vi "GearedSixMotorDriveBegin.vi"(0 "Left Rear Motor":T1=enum."Invalid", 1 "Left Middle Motor":T1=enum."Invalid", 2 "Left Front Motor":T1=enum."Invalid", 3 "Right Rear Motor":T1=enum."Invalid", 4 "Right Middle Motor":T1=enum."Invalid", 5 "Right Front Motor":T1=enum."Invalid", 8 "Left Rear Motor Inverted":bool, 9 "error in (no error)":errorcluster, 10 "Left Middle Motor Inverted":bool, 12 "Left Front Motor Inverted":bool, 14 "Right Rear Motor Inverted":bool, 16 "Right Middle Motor Inverted":bool, 18 "Right Front Motor Inverted":bool) -> (19 "error out":errorcluster, 20 "RobotDriveDevRef":T2={"DevStatus"={"status"=FALSE, "code"=0, "source"=""}, "Motors[]"=[], "Square Inputs"=FALSE, "Max Output"=1.0})   [LabVIEW 2014]
uses:
  <vilib>/Rock Robotics/SystemInterfaces/DIO/FPGA_DIOPWMChannel.ctl
  <vilib>/Rock Robotics/WPI/RobotDrive/WPI_RobotDriveDevRef.ctl
  <vilib>/Rock Robotics/WPI/MotorControl/WPI_MotorControlDeviceRef.ctl
  <vilib>/Rock Robotics/WPI/MotorControl/WPI_MotorControlType.ctl
  <vilib>/Rock Robotics/SystemInterfaces/Typedef/FPGA_TypedefDigitalModule.ctl
  <vilib>/Rock Robotics/WPI/PWM/WPI_PWMDeadband.ctl
  <vilib>/Rock Robotics/WPI/CAN/Jaguar/SubVIs/WPI_CANJaguar_ControlMode.ctl
  <vilib>/Rock Robotics/WPI/CAN/TalonSRX/WPI_CANTalonSRX_APIControlMode.ctl
  <vilib>/Rock Robotics/WPI/PWM/WPI_PWMTransform_ConPane.ctl
  <vilib>/Rock Robotics/WPI/SafetyOutput/WPI_SafetyOutputConfigMenu.ctl
  <vilib>/Rock Robotics/WPI/MotorControl/WPI_MotorControlOpenCANJaguar.vi
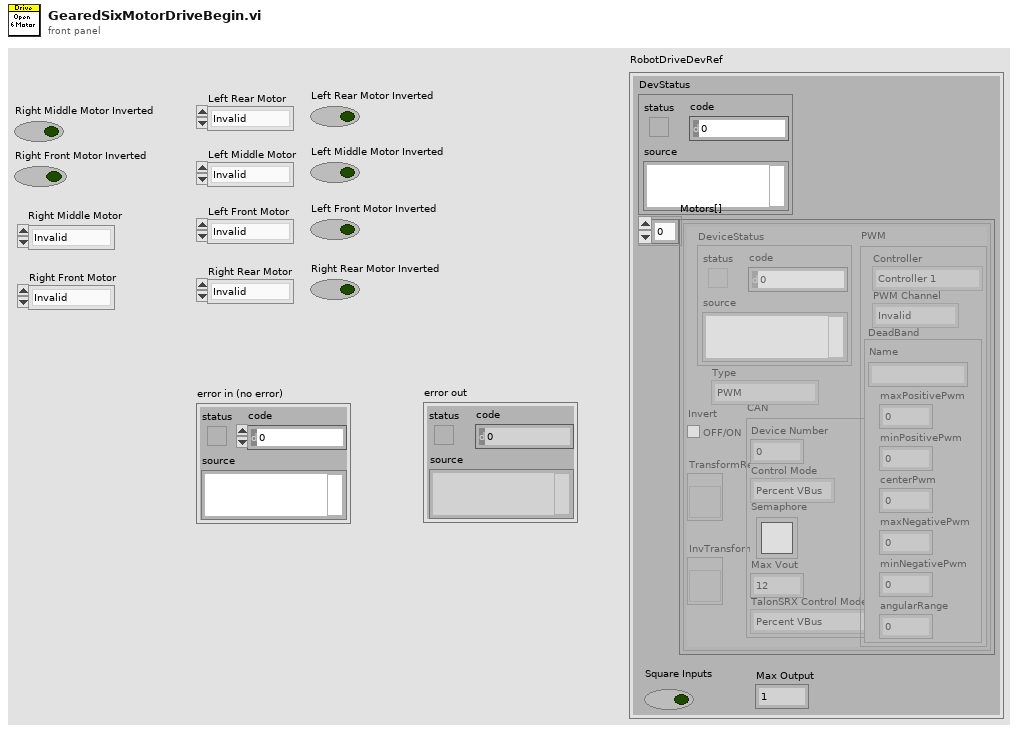
[diagram p1: front panel]
types:
  T1 = typedef "FPGA_DIOPWMChannel.ctl" = enum8{"PWM 0", "PWM 1", "PWM 2", "PWM 3", "PWM 4", "PWM 5", "PWM 6", "PWM 7", "PWM 8", "PWM 9", "PWM MXP 0", "PWM MXP 1", "PWM MXP 2", "PWM MXP 3", "PWM MXP 4", "PWM MXP 5", "PWM MXP 6", "PWM MXP 7", "PWM MXP 8", "PWM MXP 9", "Invalid"}
  T2 = typedef "WPI_RobotDriveDevRef.ctl" = cluster{"DevStatus":errorcluster, "Motors[]":T3[], "Square Inputs":bool, "Max Output":dbl}
  T3 = typedef "WPI_MotorControlDeviceRef.ctl" = cluster{"DeviceStatus":errorcluster, "Type":T4, "PWM":cluster{"Controller":T5, "PWM Channel":T1, "DeadBand":T6}, "CAN":cluster{"Device Number":u8, "Control Mode":T7, "Semaphore":T8, "Max Vout":dbl, "TalonSRX Control Mode":T9}, "Invert":bool, "TransformRef":T10, "InvTransformRef":T10}
  T4 = typedef "WPI_MotorControlType.ctl" = enum16{"PWM", "CAN", "CANTalonSRX"}
  T5 = typedef "FPGA_TypedefDigitalModule.ctl" = enum16{"Controller 1"}
  T6 = typedef "WPI_PWMDeadband.ctl" = cluster{"Name":string, "maxPositivePwm":i32, "minPositivePwm":i32, "centerPwm":i32, "maxNegativePwm":i32, "minNegativePwm":i32, "angularRange":u16}
  T7 = typedef "WPI_CANJaguar_ControlMode.ctl" = enum8{"Percent VBus", "Current", "Speed", "Position", "Voltage"}
  T8 = typedef "Semaphore RefNum" = refnum<k1>
  T9 = typedef "WPI_CANTalonSRX_APIControlMode.ctl" = enum8{"Percent VBus", "Speed", "Position", "Slave", "Unchanged / Invalid"}
  T10 = typedef "WPI_PWMTransform_ConPane.ctl" = refnum<vi>
  T11 = typedef "WPI_SafetyOutputConfigMenu.ctl" = enum16{"Enable", "Disable"}
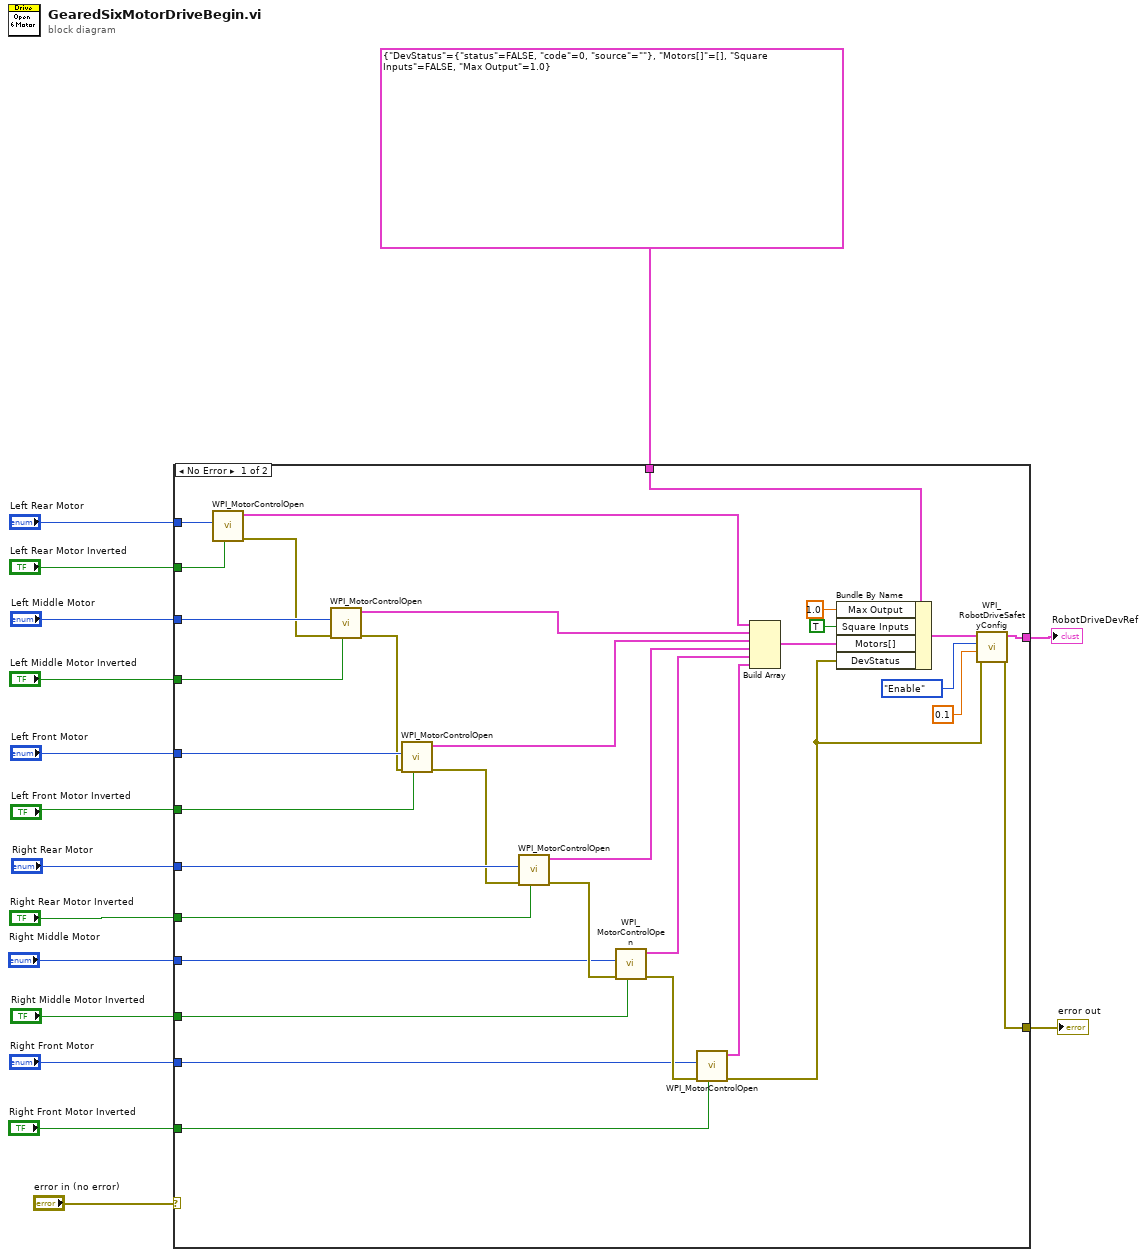
[diagram p0: block diagram]
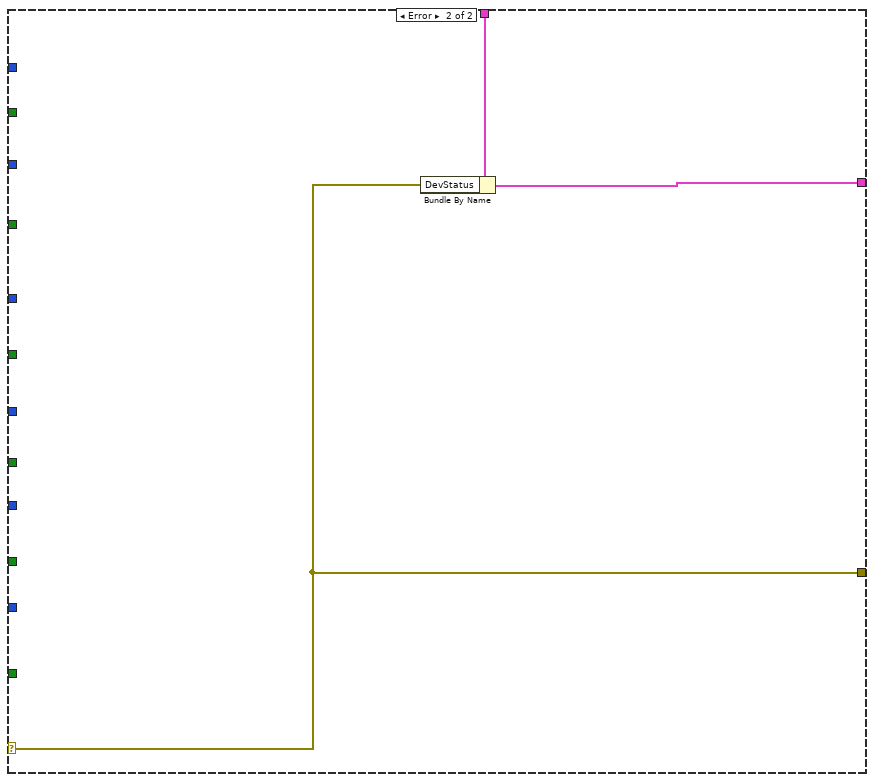
[diagram p2: hidden frame]
diagram:
  n1 = case shown="No Error" "error in (no error)" {
    selector: "error in (no error)" -> [_ w50]
    tunnel: [w30 w51] -> w16
    tunnel: T2 {"DevStatus"={"status"=FALSE, "code"=0, "source"=""}, "Motors[]"=[], "Square Inputs"=FALSE, "Max Output"=1.0} ("RobotDriveDevRef") -> [w49 w52]
    tunnel: "Left Rear Motor" -> [w47 _]
    tunnel: "Right Rear Motor" -> [w44 _]
    tunnel: "Left Front Motor" -> [w45 _]
    tunnel: "Left Middle Motor" -> [w46 _]
    tunnel: "Left Rear Motor Inverted" -> [w36 _]
    tunnel: "Left Middle Motor Inverted" -> [w35 _]
    tunnel: "Right Rear Motor Inverted" -> [w33 _]
    tunnel: "Left Front Motor Inverted" -> [w34 _]
    tunnel: [w31 w50] -> w5
    tunnel: "Right Middle Motor Inverted" -> [w20 _]
    tunnel: "Right Middle Motor" -> [w19 _]
    tunnel: "Right Front Motor" -> [w18 _]
    tunnel: "Right Front Motor Inverted" -> [w17 _]
    frame No Error {
      n2 = call-poly <vilib>:"WPI_MotorControlOpen.vi"("Invert"=w36, "Device Number"=w47) -> ("error out"=w37:errorcluster, "MotorControlDeviceRef"=w43:T3)  [unwired: 4 in, 4 out]
      n3 = call-poly <vilib>:"WPI_MotorControlOpen.vi"("Invert"=w35, "error in (no error)"=w37, "Device Number"=w46) -> ("error out"=w38:errorcluster, "MotorControlDeviceRef"=w42:T3)  [unwired: 3 in, 4 out]
      n4 = call-poly <vilib>:"WPI_MotorControlOpen.vi"("Invert"=w34, "error in (no error)"=w38, "Device Number"=w45) -> ("error out"=w39:errorcluster, "MotorControlDeviceRef"=w41:T3)  [unwired: 3 in, 4 out]
      n5 = call-poly <vilib>:"WPI_MotorControlOpen.vi"("Invert"=w33, "error in (no error)"=w39, "Device Number"=w44) -> ("error out"=w22:errorcluster, "MotorControlDeviceRef"=w40:T3)  [unwired: 3 in, 4 out]
      n6 = call-poly <vilib>:"WPI_MotorControlOpen.vi"("Invert"=w20, "error in (no error)"=w22, "Device Number"=w19) -> ("error out"=w23:errorcluster, "MotorControlDeviceRef"=w26:T3)  [unwired: 3 in, 4 out]
      n7 = call-poly <vilib>:"WPI_MotorControlOpen.vi"("Invert"=w17, "error in (no error)"=w23, "Device Number"=w18) -> ("error out"=w21:errorcluster, "MotorControlDeviceRef"=w24:T3)  [unwired: 3 in, 4 out]
      n8 = Build Array(w43, w42, w41, w40, w26, w24) -> (w25:T3[])
      n9 = Bundle By Name(cluster=w49, "Max Output"=1.0, "Square Inputs"=TRUE ("DestroyPWM?"), "Motors[]"=w25, "DevStatus"=w21) -> (w28:T2)
      n10 = call <vilib>:"WPI_RobotDriveSafetyConfig.vi"("error in (no error)"=w21, "timeout (s)"=0.1, "mode"=WPI_SafetyOutputConfigMenu."Enable", "RobotDriveDevRef"=w28) -> ("error out"=w31:errorcluster, "RobotDriveDevRef"=w30:T2)  [unwired: 6 out]
    }
    frame Error {
      n11 = Bundle By Name(cluster=w52, "DevStatus"=w50) -> (w51:T2)
    }
  }
  "RobotDriveDevRef" <- w16
  "error out" <- w5
